vi "Draw Intersections.vi"(5 "TagsArray":refnum<class "Tag.lvclass">[](array[class]), 7 "TagIDDistanceClusterArray":cluster{"TagIDTo":dbl, "Distance":dbl}[](array[cluster]), 9 "AnchorsArray":refnum<class "Anchor.lvclass">[](array[class])) -> (8 "XY Graph Out":cluster{"x":dbl[], "y":dbl[]}[](graph))   [LabVIEW 2014, in "Tag.lvclass"]
uses:
  Tag.lvclass
  Anchor/Anchor.lvclass
  Tag.lvclass/Tag.ctl
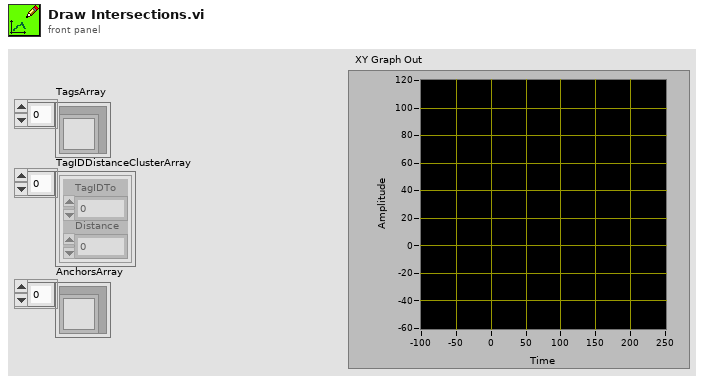
[diagram p1: front panel]
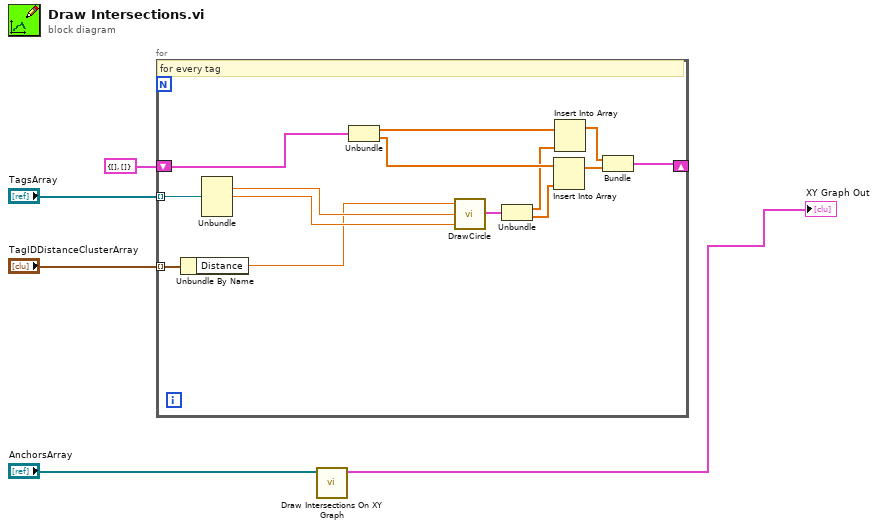
[diagram p0: block diagram]
diagram:
  n1 = for {
    tunnel: "TagsArray" -> [w19] mode=indexing
    tunnel: "TagIDDistanceClusterArray" -> [w18] mode=indexing
    shift-right: [w6] -> _
    shift-left: cluster{dbl[], dbl[]} {[], []} ("XY Graph") -> [w13]
    # "for every tag"
    n2 = Unbundle By Name(w18) -> ("Distance"=w15:dbl)
    n3 = Unbundle(w19) -> (w17:dbl, w16:dbl)  [unwired: 3 out]
    n4 = Unbundle(w13) -> (w12:dbl[], w11:dbl[])
    n5 = call "DrawCircle.vi"("y"=w16, "x"=w17, "r"=w15) -> ("XY Graph"=w14:cluster{dbl[], dbl[]})
    n6 = Unbundle(w14) -> (w10:dbl[], w9:dbl[])
    n7 = Insert Into Array(array=w11, new element=w9) -> (w7:dbl[])  [unwired: 1 in]
    n8 = Insert Into Array(array=w12, new element=w10) -> (w8:dbl[])  [unwired: 1 in]
    n9 = Bundle(w8, w7) -> (w6:cluster{dbl[], dbl[]})  [unwired: 1 in]
  }
  n10 = call "Draw Intersections On XY Graph.vi"("CombinedAnchorArray In"="AnchorsArray") -> ("XY Graph Out"=→"XY Graph Out":cluster{"x":dbl[], "y":dbl[]}[])  [unwired: 10 in]
